vi "Method_Const.vi"(4 "Boolean":bool, 5 "A":refnum<class "Abs_Boolean.lvclass">) -> (1 "Result":refnum<class "Abs_Boolean.lvclass">)   [LabVIEW 2021, in "NAND_Bool.lvclass"]
uses:
  NAND_Bool.lvclass
  Abs_Types/Boolean/Abs_Boolean.lvclass
  C:/TSA/LV_Abstract/Source/Functions/Support/Function/Two Terminal/Boolean/AbsFunc_Two Term_Bool.lvclass
  C:/Program Files (x86)/National Instruments/LabVIEW 2021/vi.lib/TSA/Abstract Data Classes/Abs_Types/Boolean/Abs_Boolean.lvclass
  Support/Function/Two Terminal/Boolean/AbsFunc_Two Term_Bool.lvclass/AbsFunc_Two Term_Bool.ctl
  Support/Function/Two Terminal/Boolean/Properties/Write Bool A.vi
  Support/Function/Two Terminal/Boolean/Properties/Write Bool B.vi
  Constants/Support/Bool/Const_Bool.lvclass
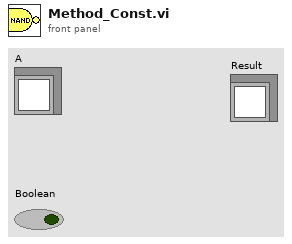
[diagram p1: front panel]
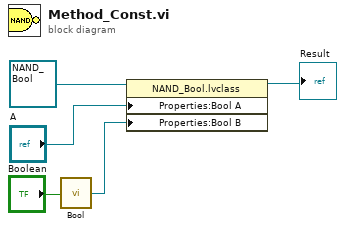
[diagram p0: block diagram]
diagram:
  n1 = call "Bool.vi"("Boolean"="Boolean") -> ("Abs_Boolean.lvclass"=w2:refnum<class "Abs_Boolean.lvclass">)  [unwired: 4 in]
  n2 = property class="NAND_Bool.lvclass"(reference=refnum<class "NAND_Bool.lvclass"> refnum ("Functions.lvlib:Logic.lvlib:AND.lvclass"), "Properties:Bool A"="A", "Properties:Bool B"=w2) -> (reference out=→"Result":refnum<class "NAND_Bool.lvclass">)  [unwired: 1 in, 1 out]
